vi "MDPtr ValidateFlattenToString4.vi"() -> ()   [LabVIEW 2017]
uses:
  <vilib>/Utility/High Resolution Relative Seconds.vi
  <vilib>/measure/NI_MABase.lvlib
panel:
  out "length 2":i32
  out "Waveform Graph 5":waveform(dbl)[](graph)
  out "Waveform Graph 4":waveform(dbl)[](graph)
  out "Waveform Graph 3":dbl[](graph)
  out "x-y 2":u32
  out "length":i32
  out "Waveform Graph 2":i32[](graph)
  out "Waveform Graph":dbl[](graph)
  out "x-y":u32
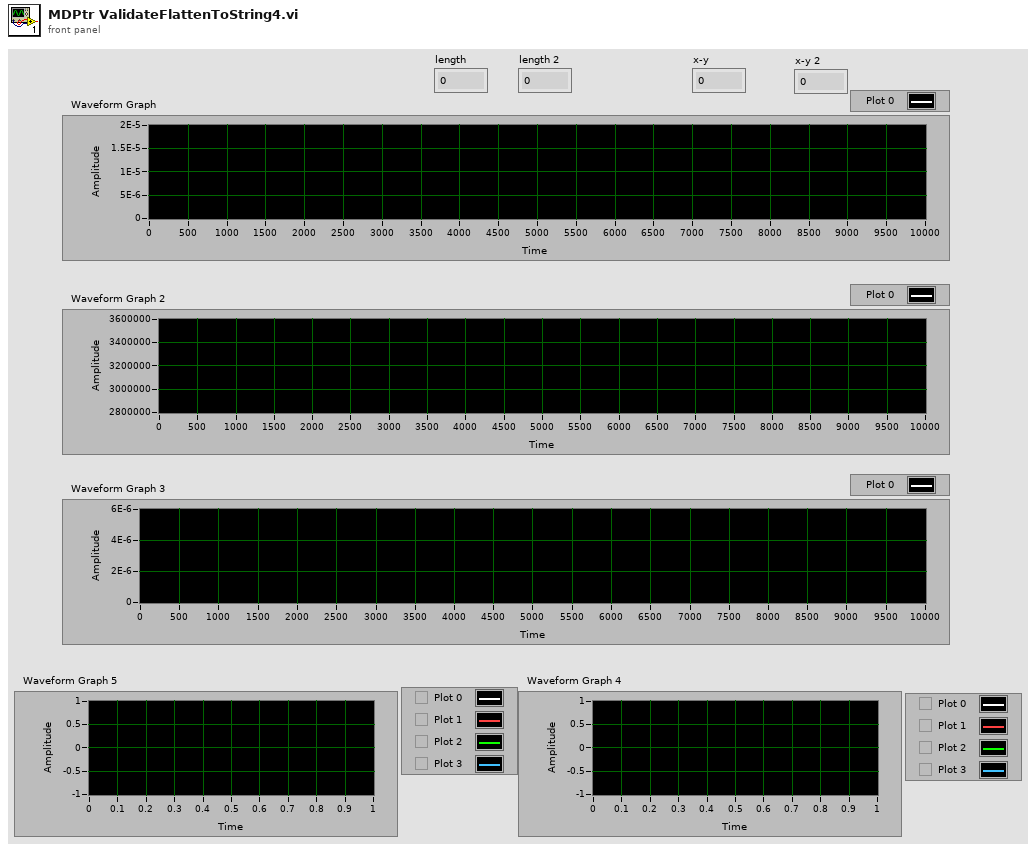
[diagram p1: front panel]
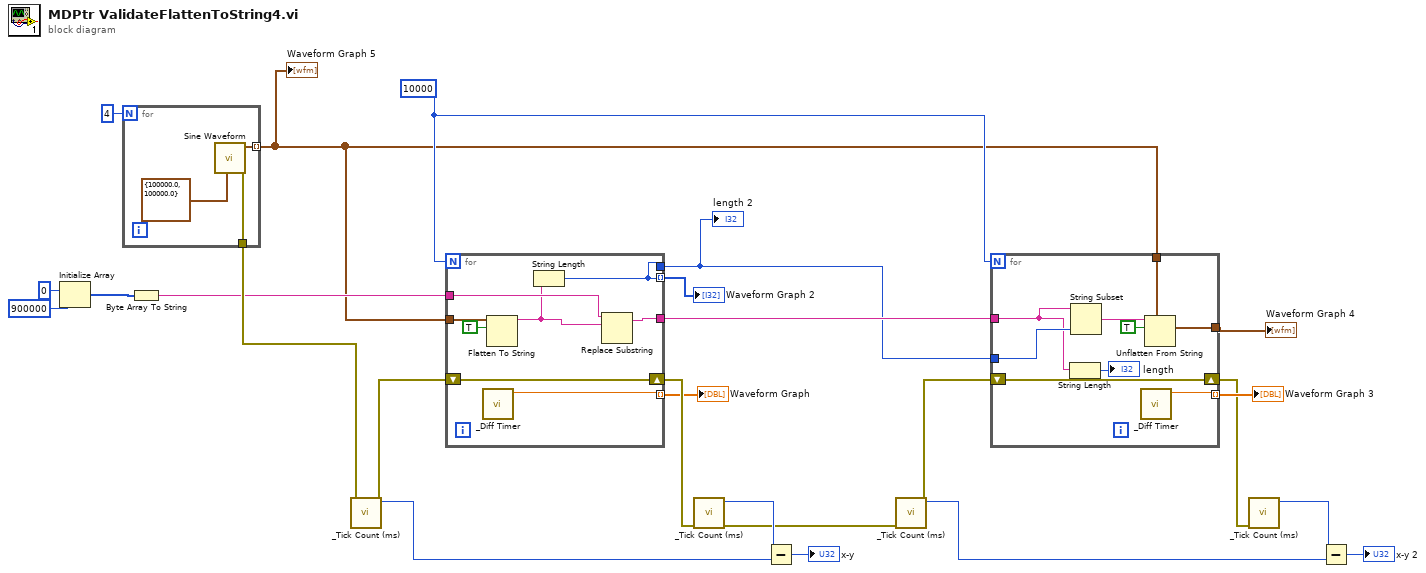
[diagram p0: block diagram]
diagram:
  w9 = 10000
  n1 = Initialize Array(u8 0 ("element"), 900000 ("dimension size")) -> (w6:u8[])
  n2 = for {
    N: 4 -> [_]
    tunnel: [w27] -> w23
    tunnel: [w26] -> w3 mode=indexing
    n3 = call <vilib>:"Sine Waveform.vi"("sampling info"=cluster{"Fs":dbl, "#s":dbl} {"Fs"=100000.0, "#s"=100000.0}) -> ("error out"=w27:errorcluster, "signal out"=w26:waveform(dbl))  [unwired: 9 in]
  }
  "Waveform Graph 5" <- w3
  n4 = Byte Array To String(unsigned byte array=w6) -> (string=w5:string)
  n5 = call "_Tick Count (ms).vi"("error in (no error)"=w23) -> ("error out"=w22:errorcluster, "millisecond timer value"=w24:u32)  [unwired: 9 in]
  n6 = for {
    N: w9 -> [_]
    tunnel: w3 -> [w36]
    tunnel: [w35] -> w19 mode=indexing
    shift-right: [w34] -> w21
    shift-left: w22 -> [w34]
    tunnel: [w30] -> w18 mode=indexing
    tunnel: [w31] -> w10
    tunnel: [w30] -> w2
    tunnel: w5 -> [w33]
    n7 = call "_Diff Timer.vi"() -> ("time diff(s)"=w35:dbl)  [unwired: 10 in, 1 out]
    n8 = Flatten To String(anything=w36, prepend array or string size? (T)=TRUE) -> (data string=w32:string)  [unwired: 2 in, 2 out]
    n9 = String Length(string=w32) -> (length=w30:i32)
    n10 = Replace Substring(4:w32, 5:w33) -> (1:w31:string)  [unwired: 2 in, 1 out]
  }
  "Waveform Graph" <- w19
  "Waveform Graph 2" <- w18
  "length 2" <- w2
  n11 = call "_Tick Count (ms).vi"("error in (no error)"=w21) -> ("error out"=w11:errorcluster, "millisecond timer value"=w25:u32)  [unwired: 9 in]
  n12 = Subtract(x=w25, y=w24) -> (x-y=→"x-y":u32)
  n13 = call "_Tick Count (ms).vi"("error in (no error)"=w11) -> ("error out"=w14:errorcluster, "millisecond timer value"=w13:u32)  [unwired: 9 in]
  n14 = for {
    N: w9 -> [_]
    tunnel: [w45] -> w17 mode=indexing
    shift-right: [w44] -> w15
    shift-left: w14 -> [w44]
    tunnel: w10 -> [w40]
    tunnel: w3 -> [w43]
    tunnel: [w42] -> w4
    tunnel: w2 -> [w41]
    n15 = String Length(string=w40) -> (length=→"length":i32)
    n16 = String Subset(string=w40, length (rest)=w41) -> (substring=w38:string)  [unwired: 1 in]
    n17 = call "_Diff Timer.vi"() -> ("time diff(s)"=w45:dbl)  [unwired: 10 in, 1 out]
    n18 = Unflatten From String(type=w43, binary string=w38, data includes array or string size? (T)=TRUE) -> (value=w42:waveform(dbl)[])  [unwired: 2 in, 2 out]
  }
  "Waveform Graph 3" <- w17
  "Waveform Graph 4" <- w4
  n19 = call "_Tick Count (ms).vi"("error in (no error)"=w15) -> ("millisecond timer value"=w12:u32)  [unwired: 9 in, 1 out]
  n20 = Subtract(x=w12, y=w13) -> (x-y=→"x-y 2":u32)
